vi "Launch and Store Client Proxy in Controller.vi"(8 "error in (no error)":errorcluster, 10 "Network Actor in":refnum<class "Client Proxy LNA.lvclass">, 11 "Server Controller in":refnum<class "Server Controller.lvclass">) -> (0 "error out":errorcluster, 3 "Server Controller Out":refnum<class "Server Controller.lvclass">)   [LabVIEW 2026, in "Server Controller.lvlib" / "Server Controller.lvclass"]
uses:
  Server Controller.lvclass
  Client Proxy LNA/Client Proxy LNA.lvclass
  C:/Users/E2013170/Documents/GitHub/Measurement-Utility-Reference/recovery/packages/ni_lib_linked_network_actor-1.2.0.19-9492AF5A82/File Group 0/vi.lib/NI/Actors/Linked Network Actor/Linked Network Actor/Linked Network Actor.lvclass
  Server Controller.lvclass/Server Controller.ctl
  recovery/packages/ni_lib_linked_network_actor-1.2.0.19-9492AF5A82/File Group 0/vi.lib/NI/Actors/Linked Network Actor/Linked Network Actor/Linked Network Actor.lvclass/Linked Network Actor.ctl
  Client Proxy LNA/Client Proxy LNA.lvclass/Client Proxy LNA.ctl
  recovery/packages/ni_lib_linked_network_actor-1.2.0.19-9492AF5A82/File Group 0/vi.lib/NI/Actors/Linked Network Actor/Linked Network Actor Messages/Connect Msg/Connect Msg.lvclass
  recovery/packages/ni_lib_linked_network_actor-1.2.0.19-9492AF5A82/File Group 0/vi.lib/NI/Actors/Linked Network Actor/Linked Network Actor/Linked Network Actor.lvclass
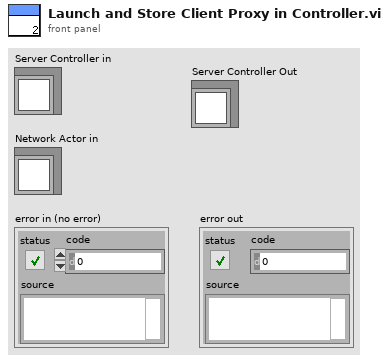
[diagram p1: front panel]
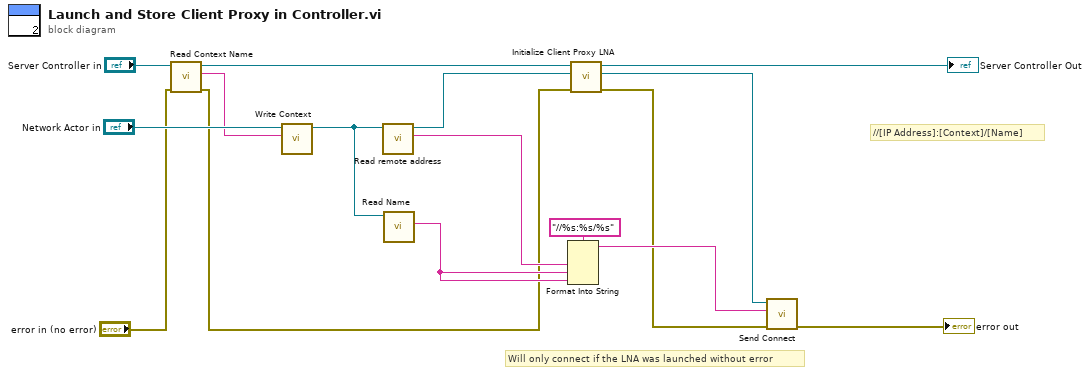
[diagram p0: block diagram]
diagram:
  # "Will only connect if the LNA was launched without error"
  # "//[IP Address]:[Context]/[Name]"
  n1 = call "Read Context Name.vi"("error in (no error)"="error in (no error)", "Server Controller in"="Server Controller in") -> ("error out"=w1:errorcluster, "Context Name"=w3:string, "Server Controller out"=w4:refnum<class "Server Controller.lvclass">)  [unwired: 7 in]
  n2 = call "Write Context.vi"("Context"=w3, "Linked Network Actor in"="Network Actor in") -> ("Linked Network Actor out"=w6:refnum<class "Client Proxy LNA.lvclass">)  [unwired: 9 in]
  n3 = call "Read remote address.vi"("Client Proxy LNA in"=w6) -> ("remote address"=w9:string, "Client Proxy LNA out"=w10:refnum<class "Client Proxy LNA.lvclass">)  [unwired: 8 in, 1 out]
  n4 = call-dynamic "Read Name.vi"("Network Actor in"=w6) -> ("Name"=w13:string)  [unwired: 10 in]
  n5 = Format Into String(format string="//%s:%s/%s" ("string"), w9, w13, w13) -> (resulting string=w14:string)  [unwired: 2 in, 1 out]
  n6 = call "Initialize Client Proxy LNA.vi"("error in (no error)"=w1, "Network Actor in"=w10, "Server Controller in"=w4) -> ("error out"=w11:errorcluster, "Caller-To-Actor Enqueuer"=w15:refnum<class "Message Enqueuer.lvclass">, "Server Controller out"=→"Server Controller Out":refnum<class "Server Controller.lvclass">)  [unwired: 6 in]
  n7 = call "Send Connect.vi"("error in (no error)"=w11, "URL"=w14, "Message Enqueuer"=w15) -> ("error out"=→"error out":errorcluster)  [unwired: 7 in, 1 out]
